vi "GetValve.vi"(1 "Numeric":i32) -> (0 "Boolean":bool)   [LabVIEW 2011]
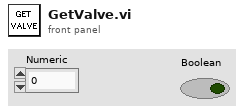
[diagram p1: front panel]
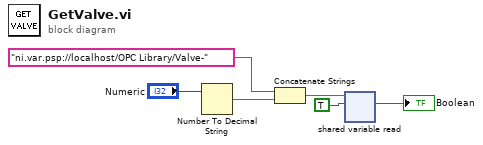
[diagram p0: block diagram]
diagram:
  n1 = Number To Decimal String(number="Numeric") -> (decimal integer string=w5:string)  [unwired: 1 in]
  n2 = Concatenate Strings("ni.var.psp://localhost/OPC Library/Valve-", w5) -> (w3:string)
  n3 = shared-variable-read(w3, TRUE) -> (→"Boolean":bool)  [unwired: 1 in, 3 out]
